vi "GetNumberPublishers.vi"(8 "error in (no error)":errorcluster, 11 "Topic Actor Descriptor in":refnum<class "Topic Actor Descriptor.lvclass">) -> (0 "error out":errorcluster, 2 "N Publishers":u32, 3 "Topic Actor Descriptor out":refnum<class "Topic Actor Descriptor.lvclass">)   [LabVIEW 2016, in "Stream Mediator.lvlib" / "Topic Actor Descriptor.lvclass"]
doc: "--\nCopyright © 2017 Composed SystemsI All rights reserved.\n\nAuthor: Jon McBee <jon.mcbee@composed.io>\n\nThis library is provided \"AS IS\" ,WITHOUT WARRANTIES OR\nCONDITIONS OF ANY KIND, either express or implied.\n\nComposed Systems -- composed.io\n\nStream 0.0.1.1\nJon McBee - Composed Systems\nCopyright (c) 2017, Composed Systems"
uses:
  <userlib>/Composed Systems/Stream/Mediator/Classes/Topic Actor Descriptor/Topic Actor Descriptor.lvclass
  <userlib>/Composed Systems/Stream/Mediator/Classes/Topic Actor Descriptor/Topic Actor Descriptor.lvclass/Topic Actor Descriptor.ctl
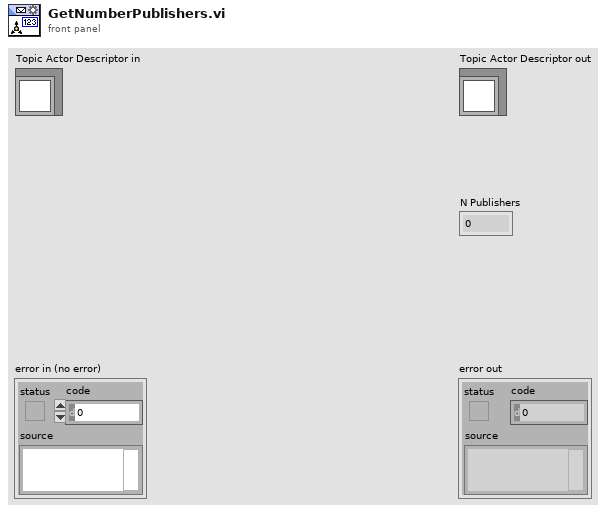
[diagram p1: front panel]
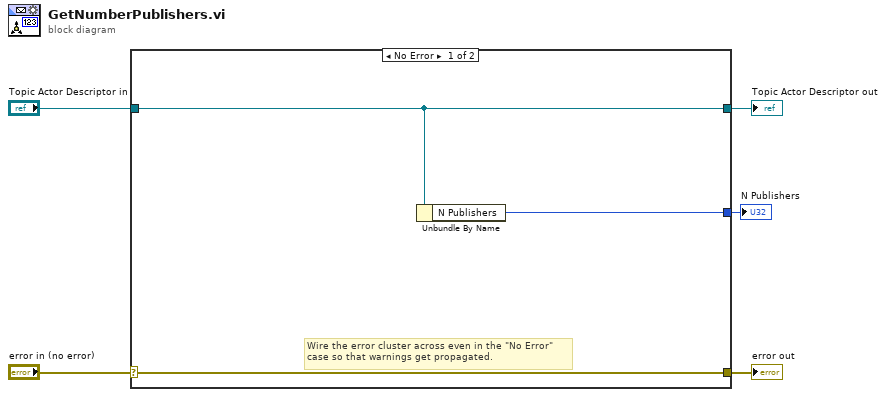
[diagram p0: block diagram]
diagram:
  n1 = case shown="No Error" "error in (no error)" {
    selector: "error in (no error)" -> [w8 w10]
    tunnel: [w8 w10] -> w4
    tunnel: [w7 w9] -> w2
    tunnel: "Topic Actor Descriptor in" -> [w7 w9]
    tunnel: [w6 _] -> w1
    frame No Error {
      # "Wire the error cluster across even in the \"No Error\"\ncase so that warnings get propagated."
      n2 = Unbundle By Name(w7) -> ("N Publishers"=w6:u32)
    }
    frame Error {
    }
  }
  "error out" <- w4
  "Topic Actor Descriptor out" <- w2
  "N Publishers" <- w1
